vi "ReadAllRegisters.vi"(8 "error in (no error)":errorcluster, 11 "Serial Config":T1={"设备名称"="", "串口选择"="COM1", "仪器地址"=200, "通讯速率"=8, "超时时间"=0, "刷新时间"=10.0}) -> (0 "error out":errorcluster, 3 "AllRegisterData":i16[](array[numeric]))   [LabVIEW 2010, in "MonitorServer.lvlib"]
uses:
  MonitorServer.lvlib
  Serial Config.ctl
panel:
  out "Array":errorcluster[](array[cluster])
  out "Numeric":i32
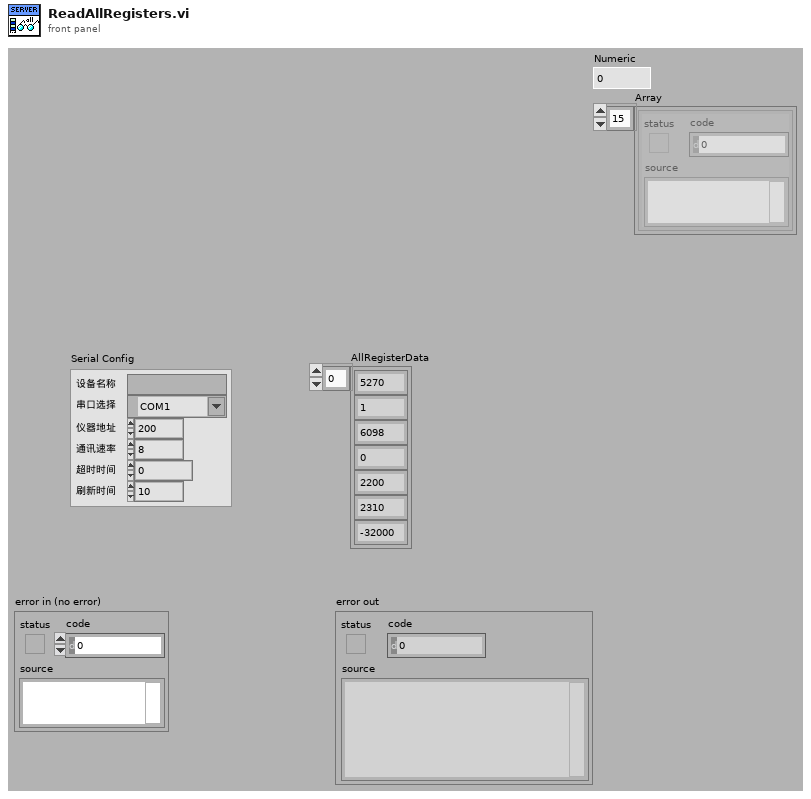
[diagram p1: front panel]
types:
  T1 = typedef "MonitorServer.lvlib/Serial Config.ctl" = cluster{"设备名称":string, "串口选择":refnum<visa-resource-name>, "仪器地址":u32, "通讯速率":u32, "超时时间":u32, "刷新时间":dbl}
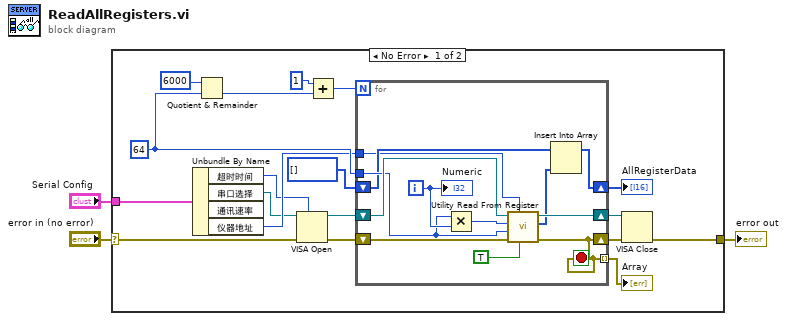
[diagram p0: block diagram]
diagram:
  n1 = case shown="No Error" "error in (no error)" {
    selector: "error in (no error)" -> [w4 w34]
    tunnel: "Serial Config" -> [w21 _]
    tunnel: [w10 w34] -> w1
    frame No Error {
      w16 = u16 64 ("Num Of Reg (1)")
      n2 = Unbundle By Name(w21) -> ("超时时间"=w7:u32, "串口选择"=w8:refnum<visa-resource-name>, "仪器地址"=w11:u32)  [unwired: 1 out]
      n3 = Quotient & Remainder(x=u16 6000, y=w16) -> (floor(x/y)=w19:u16)  [unwired: 1 out]
      n4 = VISA Open(timeout (0)=w7, error in (no error)=w4, VISA resource name=w8) -> (VISA resource name=w6:refnum<visa-resource-name>, error out=w5:errorcluster)  [unwired: 2 in]
      n5 = Add(x=u16 1, y=w19) -> (x+y=w18:u16)
      n6 = for {
        N: w18 -> [_]
        tunnel: w16 -> [w30]
        shift-right: [w25] -> w13
        shift-left: i16[] [] -> [w24]
        shift-right: [w22] -> w12
        shift-left: w5 -> [w28]
        shift-right: [w27] -> w15
        shift-left: w6 -> [w32]
        tunnel: w11 -> [w23]
        tunnel: [w22] -> w9 mode=indexing
        i -> [w31]
        stop <- w22 stop-if-true
        n7 = Multiply(x=w30, y=w31) -> (x*y=w29:i32)
        n8 = call "Utility Read From Register.vi"("Direct Action?"=TRUE, "Unit Address (1)"=w23, "error in (no error)"=w28, "Num Of Reg (1)"=w30, "Register Address (0)"=w29, "VISA resource name"=w32) -> ("error out"=w22:errorcluster, "Data"=w26:i16[], "VISA resource name out"=w27:refnum<visa-resource-name>)  [unwired: 3 in]
        n9 = Insert Into Array(array=w24, new element=w26) -> (w25:i16[])  [unwired: 1 in]
        "Numeric" <- w31
      }
      "AllRegisterData" <- w13
      "Array" <- w9
      n10 = VISA Close(VISA resource name=w15, error in (no error)=w12) -> (error out=w10:errorcluster)
    }
    frame Error {
    }
  }
  "error out" <- w1
